vi "test8-AsteriskWildcardStatusRegistration.vi"(8 "error in (no error)":errorcluster, 11 "TestCase in":refnum<class "testcase-CSMStatusStateRegisterUnregister.lvclass">) -> (0 "error out":errorcluster, 3 "TestCase out":refnum<class "testcase-CSMStatusStateRegisterUnregister.lvclass">)   [LabVIEW 2017, in "testcase-CSMStatusStateRegisterUnregister.lvclass"]
uses:
  testcase-CSMStatusStateRegisterUnregister.lvclass
  0c20cacf-7d77-4f8e-aec5-f22e7d09936d.vi
  26de337d-8090-412f-9da5-e117a55d4726.vi
  de10340a-d592-45ad-b055-7fa7b377c551.vi
  e3eae2f8-d8ce-4adb-8167-9a417250fce1.vi
  a4d00e00-a9ed-4631-bf53-269bf71f16fc.vi
  src/user.lib/_NEVSTOP/Communicable State Machine(CSM)/AdvanceAPI/CSM - Revert Arguments-Safe String.vi
  src/user.lib/_NEVSTOP/Communicable State Machine(CSM)/AdvanceAPI/CSM - Make String Arguments Safe.vi
  src/user.lib/_NEVSTOP/Communicable State Machine(CSM)/AdvanceAPI/CSM - Break Down Multiple States String.vi
  src/user.lib/_NEVSTOP/Communicable State Machine(CSM)/AdvanceAPI/CSM - Compact Multiple States.vi
  src/user.lib/_NEVSTOP/Communicable State Machine(CSM)/AdvanceAPI/CSM - Keywords.vi
  src/user.lib/_NEVSTOP/Communicable State Machine(CSM)/_Shared/Trim Single-line Text.vi
  src/user.lib/_NEVSTOP/Communicable State Machine(CSM)/AdvanceAPI/CSM - Set Module Attribute.vi
  src/user.lib/_NEVSTOP/Communicable State Machine(CSM)/AdvanceAPI/CSM - Get Module Attribute.vi
  <vilib>/addons/_JKI Toolkits/VI Tester/TestCase.llb/TestCase.lvclass
  src/user.lib/_NEVSTOP/Communicable State Machine(CSM)/Communicable State Machine.lvlib
  C:/Program Files (x86)/National Instruments/LabVIEW 2017/vi.lib/addons/_JKI Toolkits/VI Tester/TestCase.llb/TestCase.lvclass
panel:
  out "error out 2":errorcluster
  out "Execution Times":i32
  out "State History":string
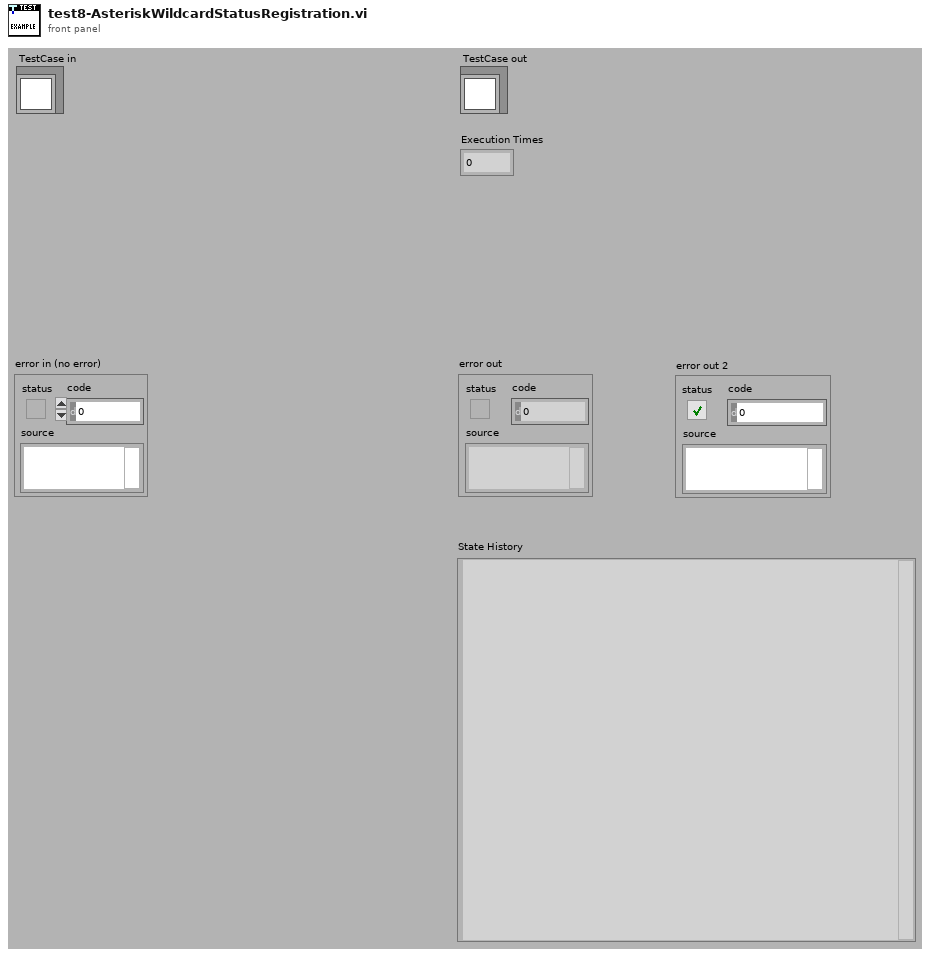
[diagram p1: front panel]
types:
  T1 = enum32{"Invalid", "Standard", "Closed", "Hidden", "Minimized", "Maximized"}
  T2 = enum32{"invalid app kind", "Development System", "Run Time System", "Student Edition", "Embedded LabVIEW", "Evaluation", "Custom"}
  T3 = typedef "Communicable State Machine.lvlib/_CSM_Response Source Message.ctl" = cluster{"‘State":string, "’Arguments":string, "’Error":errorcluster}
  T4 = cluster{"Current VI Reference":refnum<vi>, "Close Panel on Exit?":bool}
  T5 = cluster{"Core":cluster{"Current VI Reference":refnum<vi>, "Close Panel on Exit?":bool}, "Your Boolean data":bool, "Your string data":string, "TestData":i32}
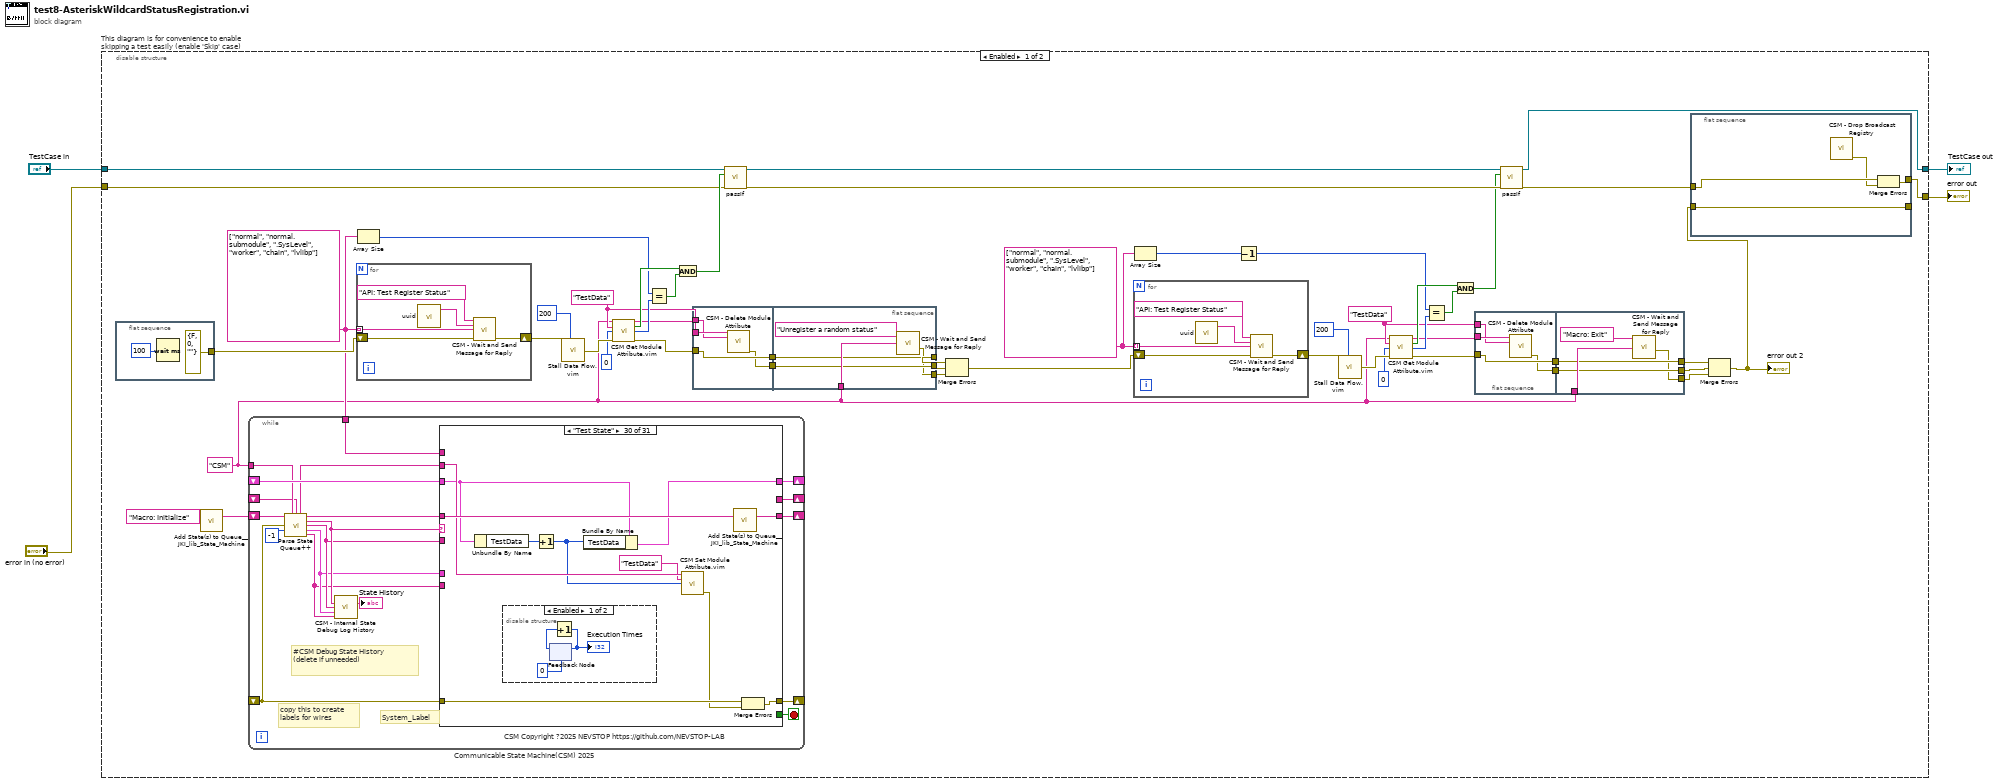
[diagram p0: block diagram]
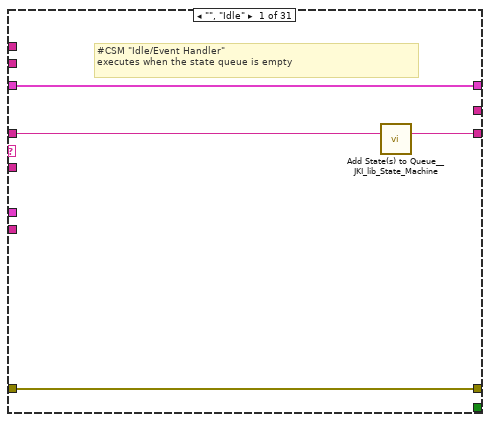
[diagram p2: hidden frame]
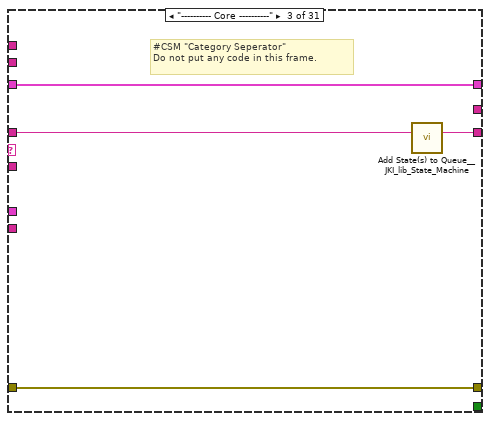
[diagram p4: hidden frame]
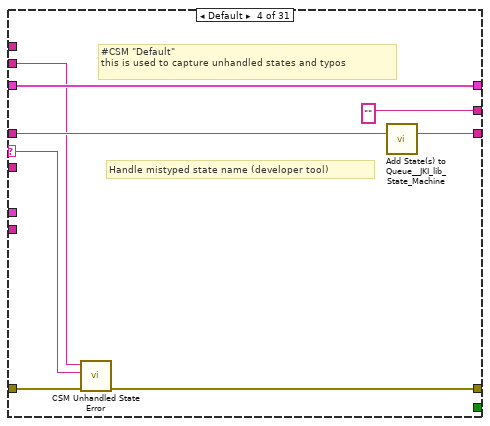
[diagram p5: hidden frame]
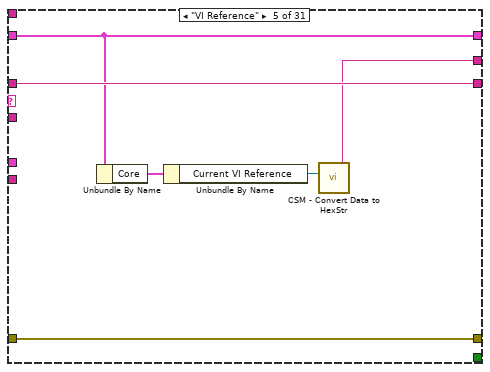
[diagram p6: hidden frame]
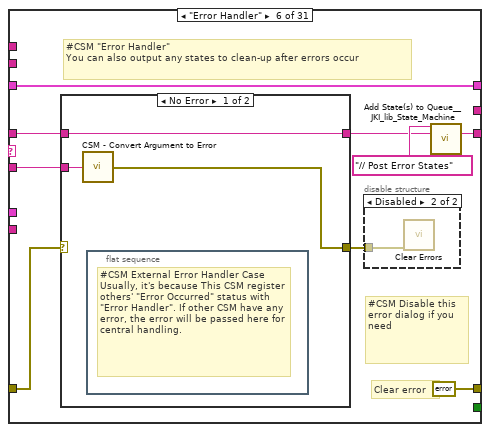
[diagram p7: hidden frame]
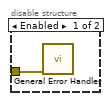
[diagram p8: hidden frame]
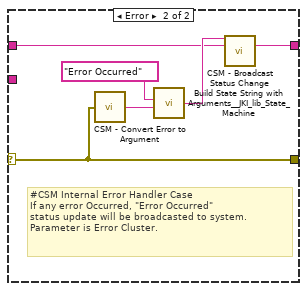
[diagram p9: hidden frame]
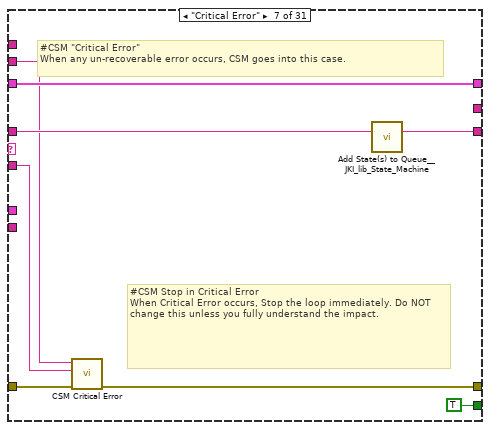
[diagram p10: hidden frame]
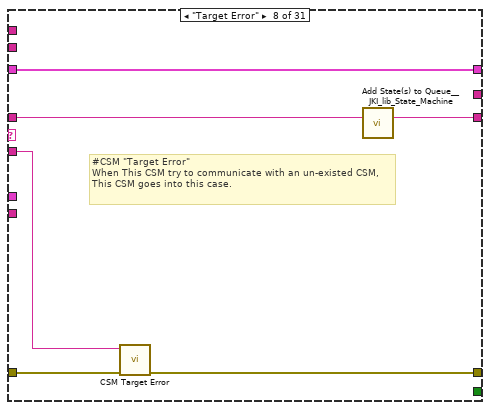
[diagram p11: hidden frame]
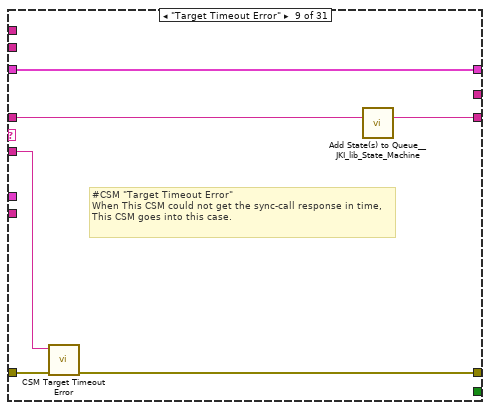
[diagram p12: hidden frame]
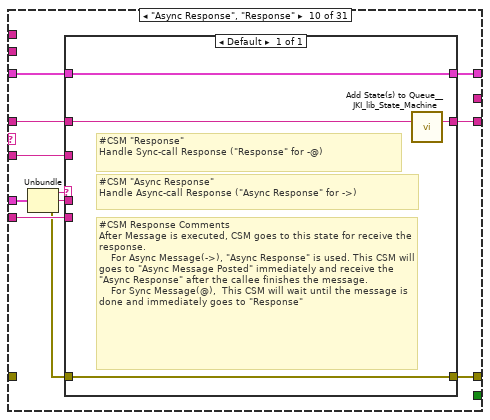
[diagram p13: hidden frame]
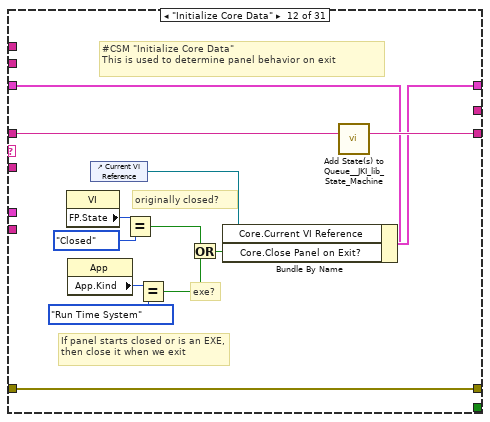
[diagram p15: hidden frame]
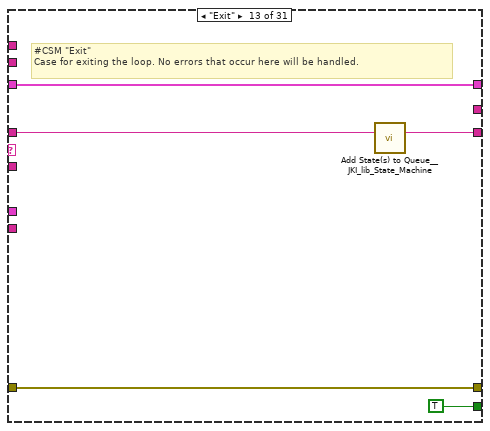
[diagram p16: hidden frame]
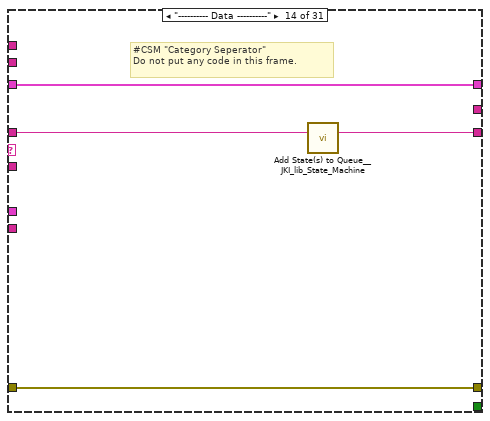
[diagram p17: hidden frame]
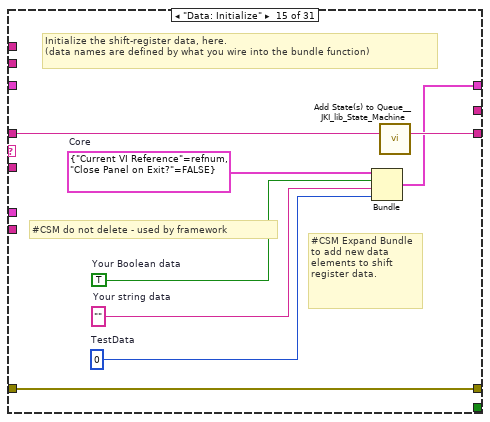
[diagram p18: hidden frame]
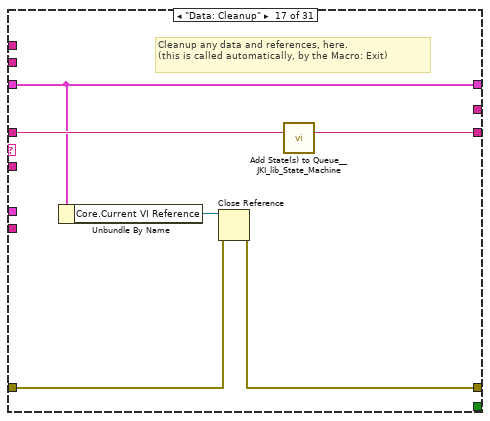
[diagram p20: hidden frame]
diagram:
  n1 = disable-structure "This diagram is for convenience to enable skipping a test easily (enable 'Skip' case)" shown="Enabled" {
    disable-tunnel: "TestCase in" -> [w41 w408]
    disable-tunnel: [w16 w406] -> w1
    disable-tunnel: [w52 w407] -> w3
    disable-tunnel: "error in (no error)" -> [w40 w405]
    frame Enabled {
      w12 = "TestData" ("Attribute")
      w23 = string[] ["normal", "normal.submodule", ".SysLevel", "worker", "chain", "lvlibp"]
      w38 = "TestData" ("Attribute")
      w10 = "CSM" ("Name (\"\" to Use UUID)")
      w31 = string[] ["normal", "normal.submodule", ".SysLevel", "worker", "chain", "lvlibp"]
      n2 = flat-sequence {
        tunnel: [errorcluster {"status"=FALSE, "code"=0, "source"=""} ("error in (no error)")] -> w51
        frame #0 {
          n3 = Wait (ms)(milliseconds to wait=u32 100) -> ()  [unwired: 1 out]
        }
      }
      n4 = call <vilib>:"Add State(s) to Queue__JKI_lib_State_Machine.vi"("State(s) in (\"\")"="Macro: Initialize" ("Init State(\"Macro: Initialize\")")) -> ("States Out"=w53:string)  [unwired: 14 in]
      n5 = while "Communicable State Machine(CSM) 2025" {
        shift-right: [w97] -> _
        shift-left: _ -> [w96]
        shift-right: [w100] -> _
        shift-left: _ -> [w95]
        shift-right: [w99] -> _
        shift-left: w53 -> [w101]
        tunnel: w10 -> [w93]
        shift-right: [w94] -> _
        shift-left: _ -> [w87]
        tunnel: w31 -> [w84]
        stop <- w98 stop-if-true
        # "#CSM Debug State History\n(delete if unneeded)"
        # "copy this to create labels for wires"
        # "System_Label"
        # "CSM Copyright ?2025 NEVSTOP https://github.com/NEVSTOP-LAB"
        n6 = call "Parse State Queue++.vi"("State Queue"=w101, "Name (\"\" to Use UUID)"=w93, "Response Arguments"=w87, "Previous Error"=w95, "Dequeue (1 ms)"=-1 ("Timeout")) -> ("Name Used"=w88:string, "Remaining States"=w102:string, "Current State"=w92:string, "Arguments"=w91:string, "Additional Information"=w90:T3, "Source CSM"=w89:string)  [unwired: 5 in]
        n7 = call "CSM - Internal State Debug Log History.vi"("State"=w92, "Arguments (\"\")"=w91, ">> Response Source Message >>"=w90, "Source (\"\")"=w89) -> ("Debug Log"=→"State History":string)  [unwired: 11 in]
        n8 = case shown="\"Test State\"" w92 {
          selector: w92 -> [_ _ _ w116 _ _ _ _ _ _ _ _ _ _ _ _ _ _ _ _ _ _ _ _ _ _ _ _ _ _ _]
          tunnel: w102 -> [w103 w108 w113 w120 w126 w132 w153 w159 w165 w173 w184 w198 w203 w207 w215 w217 w224 w228 w232 w238 w253 w322 w333 w346 w348 w352 w357 w364 w368 w379 w399]
          tunnel: w91 -> [_ _ _ _ _ w131 w149 w158 w163 w172 _ _ _ _ _ _ _ _ _ w233 w247 _ _ _ _ _ w355 _ _ _ _]
          tunnel: w96 -> [w104 w107 w110 w118 w125 w135 w154 w160 w166 w175 w183 w191 w201 w204 _ w216 w219 w225 w230 w236 w249 w319 w330 w343 w347 w351 w356 w361 w365 w371 w385]
          tunnel: [w105 w109 w111 w114 w127 errorcluster {"status"=FALSE, "code"=0, "source"=""} ("error out") w150 w156 w162 w178 w185 w195 w200 w205 w212 w218 w220 w226 w229 w234 w250 w320 w324 w335 w349 w353 w358 w362 w366 w373 w387] -> w100
          tunnel: w95 -> [w105 w109 w111 w121 w127 w133 w155 w157 w164 _ w185 w195 w200 w205 w212 w218 w221 w226 w229 w235 w251 w320 w331 w344 w349 w353 w358 w362 w366 w377 w397]
          tunnel: [w106 w108 w112 w119 w126 w128 w152 w161 w167 w174 w184 w197 w202 w206 w214 w217 w223 w227 w231 w237 w252 w321 w332 w345 w348 w352 w357 w363 w367 w378 w398] -> w99
          tunnel: [_ _ _ _ _ _ TRUE _ _ _ _ _ TRUE _ _ _ _ _ _ _ _ _ _ _ _ _ _ _ _ _ _] -> w98
          tunnel: [w104 w107 w110 w118 w125 w135 w154 w160 w166 w176 w183 w196 w201 w204 w213 w216 w219 w225 w230 w236 w249 w319 w330 w343 w347 w351 w356 w361 w365 w375 w383] -> w97
          tunnel: w89 -> [_ _ _ _ _ _ _ _ _ w170 _ _ _ _ _ _ _ _ _ _ _ _ _ _ _ _ _ _ _ _ _]
          tunnel: w90 -> [_ _ _ _ _ _ _ _ _ w177 _ _ _ _ _ _ _ _ _ _ _ _ _ _ _ _ _ _ _ _ _]
          tunnel: [_ _ _ "" w122 _ _ _ _ _ _ _ _ _ _ _ _ _ _ _ _ _ _ _ _ "API1 Response" w354 _ _ _ _] -> w94
          tunnel: w88 -> [_ _ _ w115 _ _ w148 _ _ _ _ _ _ _ _ _ _ _ _ _ _ _ w325 w337 _ _ _ _ _ w374 w394]
          tunnel: w84 -> [_ _ _ _ _ _ _ _ _ _ _ _ _ _ _ _ _ _ _ _ _ _ _ _ _ _ _ _ _ _ w390]
          frame "", "Idle" {
            # "#CSM \"Idle/Event Handler\"\nexecutes when the state queue is empty"
            n9 = call <vilib>:"Add State(s) to Queue__JKI_lib_State_Machine.vi"("State(s) in (\"\")"=w103) -> ("States Out"=w106:string)  [unwired: 14 in]
          }
          frame "CSM Documentation" {
            # "#CSM README FIRST\n\nCommunicable State Machine(CSM) is a LabVIEW application framework that builds upon JKI State Machine(JKISM). It follows the pattern of JKISM and extends the keywords to describe message communication between modules, including concepts such as Sync-Message, Async-Message, Subscription/Unsubscription of status - essential elements for creating reusable code modules. For more information, please visit the CSM wiki: https://nevstop-lab.github.io/CSM-Wiki/\n\nFor instructions on JKI State Machine, visit: http://jki.net/state-machine/\nFor information about CSM, visit: https://github.com/NEVSTOP-LAB"
            # "#CSM \"Documentation\"\nCase for holding CSM Documenation"
          }
          frame "---------- Core ----------" {
            # "#CSM \"Category Seperator\"\nDo not put any code in this frame."
            n10 = call <vilib>:"Add State(s) to Queue__JKI_lib_State_Machine.vi"("State(s) in (\"\")"=w113) -> ("States Out"=w112:string)  [unwired: 14 in]
          }
          frame Default {
            # "#CSM \"Default\"\nthis is used to capture unhandled states and typos"
            # "Handle mistyped state name (developer tool)"
            n11 = call "CSM Unhandled State Error.vi"("error in (no error)"=w121, "Undefined State"=w116, "CSM Name"=w115) -> ("error out"=w114:errorcluster)  [unwired: 8 in]
            n12 = call <vilib>:"Add State(s) to Queue__JKI_lib_State_Machine.vi"("State(s) in (\"\")"=w120) -> ("States Out"=w119:string)  [unwired: 14 in]
          }
          frame "VI Reference" {
            n13 = Unbundle By Name(w125) -> ("Core"=w124:T4)
            n14 = Unbundle By Name(w124) -> ("Current VI Reference"=w123:refnum<vi>)
            n15 = call "CSM - Convert Data to HexStr.vi"("Variant"=w123) -> ("HEX String (0-9,A-F)"=w122:string)  [unwired: 8 in]
          }
          frame "Error Handler" {
            # "#CSM Disable this error dialog if you need"
            # "#CSM \"Error Handler\"\nYou can also output any states to clean-up after errors occur"
            # "Clear error"
            n16 = case shown="No Error" w133 {
              selector: w133 -> [_ w142]
              tunnel: [w141 w144] -> w129
              tunnel: w132 -> [w141 w143]
              tunnel: w131 -> [w140 _]
              tunnel: [w139 w142] -> w134
              frame No Error {
                n17 = call "CSM - Convert Argument to Error.vi"("Argument"=w140) -> ("Error"=w139:errorcluster)  [unwired: 4 in]
                n18 = flat-sequence {
                  frame #0 {
                    # "#CSM External Error Handler Case\nUsually, it's because This CSM register others' \"Error Occurred\" status with \"Error Handler\". If other CSM have any error, the error will be passed here for central handling."
                  }
                }
              }
              frame Error {
                # "#CSM Internal Error Handler Case \nIf any error Occurred, \"Error Occurred\" \nstatus update will be broadcasted to system.\nParameter is Error Cluster."
                n19 = call "CSM - Convert Error to Argument.vi"("Error"=w142) -> ("Argument"=w146:string)  [unwired: 4 in]
                n20 = call <vilib>:"Build State String with Arguments__JKI_lib_State_Machine.vi"("Arguments (\"\")"=w146, "State"="Error Occurred" ("Status with Arguments")) -> ("State with Arguments"=w145:string)  [unwired: 4 in]
                n21 = call "CSM - Broadcast Status Change.vi"("Status With Arguments"=w145, "State Queue"=w143) -> ("Remaining States"=w144:string)  [unwired: 13 in]
              }
            }
            n22 = disable-structure shown="Disabled" {
              disable-tunnel: w134 -> [w137 w138]
              frame Enabled {
                n23 = call <vilib>:"General Error Handler.vi"("error in (no error)"=w137) -> ()  [unwired: 10 in, 5 out]
              }
              frame Disabled {
                n24 = call <vilib>:"Clear Errors.vi"("error in (no error)"=w138) -> ()  [unwired: 5 in, 2 out]
              }
            }
            n25 = call <vilib>:"Add State(s) to Queue__JKI_lib_State_Machine.vi"("State(s) in Front (\"\")"="// Post Error States", "State(s) in (\"\")"=w129) -> ("States Out"=w128:string)  [unwired: 13 in]
          }
          frame "Critical Error" {
            # "#CSM Stop in Critical Error\nWhen Critical Error occurs, Stop the loop immediately. Do NOT change this unless you fully understand the impact."
            # "#CSM \"Critical Error\"\nWhen any un-recoverable error occurs, CSM goes into this case."
            n26 = call "CSM Critical Error.vi"("error in (no error)"=w155, "Arugments (As Reason)"=w149, "CSM Name"=w148) -> ("error out"=w150:errorcluster)  [unwired: 8 in]
            n27 = call <vilib>:"Add State(s) to Queue__JKI_lib_State_Machine.vi"("State(s) in (\"\")"=w153) -> ("States Out"=w152:string)  [unwired: 14 in]
          }
          frame "Target Error" {
            # "#CSM \"Target Error\"\nWhen This CSM try to communicate with an un-existed CSM, This CSM goes into this case."
            n28 = call "CSM Target Error.vi"("error in (no error)"=w157, "Arguments (As CSM Name)"=w158) -> ("error out"=w156:errorcluster)  [unwired: 9 in]
            n29 = call <vilib>:"Add State(s) to Queue__JKI_lib_State_Machine.vi"("State(s) in (\"\")"=w159) -> ("States Out"=w161:string)  [unwired: 14 in]
          }
          frame "Target Timeout Error" {
            # "#CSM \"Target Timeout Error\"\nWhen This CSM could not get the sync-call response in time, This CSM goes into this case."
            n30 = call "CSM Target Timeout Error.vi"("error in (no error)"=w164, "Arguments (As CSM Name)"=w163) -> ("error out"=w162:errorcluster)  [unwired: 9 in]
            n31 = call <vilib>:"Add State(s) to Queue__JKI_lib_State_Machine.vi"("State(s) in (\"\")"=w165) -> ("States Out"=w167:string)  [unwired: 14 in]
          }
          frame "Async Response", "Response" {
            n32 = Unbundle(w177) -> ("‘State"=w171:string, "’Arguments"=w169:string, "’Error"=w168:errorcluster)
            n33 = case shown="Default" w171 {
              tunnel: [w182] -> w178
              tunnel: w168 -> [w182]
              tunnel: [w181] -> w176
              tunnel: w175 -> [w181]
              tunnel: [w179] -> w174
              tunnel: w173 -> [w180]
              tunnel: w172 -> [_]
              tunnel: w170 -> [_]
              tunnel: w169 -> [_]
              frame Default {
                # "#CSM Response Comments\nAfter Message is executed, CSM goes to this state for receive the response.\n    For Async Message(->), \"Async Response\" is used. This CSM will goes to \"Async Message Posted\" immediately and receive the \"Async Response\" after the callee finishes the message.\n    For Sync Message(@),  This CSM will wait until the message is done and immediately goes to \"Response\""
                # "#CSM \"Async Response\"\nHandle Async-call Response (\"Async Response\" for ->)"
                # "#CSM \"Response\"\nHandle Sync-call Response (\"Response\" for -@)"
                n34 = call <vilib>:"Add State(s) to Queue__JKI_lib_State_Machine.vi"("State(s) in (\"\")"=w180) -> ("States Out"=w179:string)  [unwired: 14 in]
              }
            }
          }
          frame "Async Message Posted" {
            # "#CSM \"Async Message Posted\"\nAfter Async Message is posted (-> or ->| ), CSM goes to this state for post-action.\nYou can use Argument - State to tell which Async Message is called."
          }
          frame "Initialize Core Data" {
            # "#CSM \"Initialize Core Data\"\nThis is used to determine panel behavior on exit"
            # "originally closed?"
            # "exe?"
            # "If panel starts closed or is an EXE, then close it when we exit"
            n35 = property class="VI"() -> ("FP.State"=w188:T1)  [unwired: 2 in, 2 out]
            n36 = property class="App"() -> ("App.Kind"=w194:T2)  [unwired: 2 in, 2 out]
            n37 = control-ref of="Current VI Reference"() -> (w189:refnum<vi>)
            n38 = Equal?(x=w188, y=T1."Closed" ("Front Panel Window:State")) -> (x = y?=w186:bool)
            n39 = Equal?(x=w194, y=T2."Run Time System" ("Application:Kind")) -> (x = y?=w192:bool)
            n40 = Or(x=w186, y=w192) -> (x .or. y?=w190:bool)
            n41 = Bundle By Name(cluster=w191, "Core.Current VI Reference"=w189, "Core.Close Panel on Exit?"=w190) -> (w196:T5)
            n42 = call <vilib>:"Add State(s) to Queue__JKI_lib_State_Machine.vi"("State(s) in (\"\")"=w198) -> ("States Out"=w197:string)  [unwired: 14 in]
          }
          frame "Exit" {
            # "#CSM \"Exit\"\nCase for exiting the loop. No errors that occur here will be handled."
            n43 = call <vilib>:"Add State(s) to Queue__JKI_lib_State_Machine.vi"("State(s) in (\"\")"=w203) -> ("States Out"=w202:string)  [unwired: 14 in]
          }
          frame "---------- Data ----------" {
            # "#CSM \"Category Seperator\"\nDo not put any code in this frame."
            n44 = call <vilib>:"Add State(s) to Queue__JKI_lib_State_Machine.vi"("State(s) in (\"\")"=w207) -> ("States Out"=w206:string)  [unwired: 14 in]
          }
          frame "Data: Initialize" {
            w208 = 0  # TestData
            w209 = T4 {"Current VI Reference"=refnum, "Close Panel on Exit?"=FALSE}  # Core
            w211 = TRUE  # Your Boolean data
            w210 = ""  # Your string data
            # "#CSM do not delete - used by framework"
            # "#CSM Expand Bundle to add new data elements to shift register data."
            # "Initialize the shift-register data, here.\n(data names are defined by what you wire into the bundle function)"
            n45 = Bundle("Core"=w209, "Your Boolean data"=w211, "Your string data"=w210, "TestData"=w208) -> (w213:T5)  [unwired: 1 in]
            n46 = call <vilib>:"Add State(s) to Queue__JKI_lib_State_Machine.vi"("State(s) in (\"\")"=w215) -> ("States Out"=w214:string)  [unwired: 14 in]
          }
          frame "Data: Update Indicators" {
          }
          frame "Data: Cleanup" {
            # "Cleanup any data and references, here.\n(this is called automatically, by the Macro: Exit)"
            n47 = Unbundle By Name(w219) -> ("Core.Current VI Reference"=w222:refnum<vi>)
            n48 = Close Reference(reference=w222, error in (no error)=w221) -> (error out=w220:errorcluster)
            n49 = call <vilib>:"Add State(s) to Queue__JKI_lib_State_Machine.vi"("State(s) in (\"\")"=w224) -> ("States Out"=w223:string)  [unwired: 14 in]
          }
          frame "---------- UI ----------" {
            # "#CSM \"Category Seperator\"\nDo not put any code in this frame."
            n50 = call <vilib>:"Add State(s) to Queue__JKI_lib_State_Machine.vi"("State(s) in (\"\")"=w228) -> ("States Out"=w227:string)  [unwired: 14 in]
          }
          frame "UI: Initialize" {
            # "#CSM \"UI: Initialize\"\nInitialize the User Interface, here.\n(this is called automatically, by the Macro: Init)"
            n51 = call <vilib>:"Add State(s) to Queue__JKI_lib_State_Machine.vi"("State(s) in (\"\")"=w232) -> ("States Out"=w231:string)  [unwired: 14 in]
          }
          frame "UI: Cursor Set" {
            # "#CSM \"UI: Cursor Set\"\nSet and Unset Cursor Busy.\n(Usage: \"UI: Cursor Set >> Busy|Idle\")"
            # "Argument"
            n52 = disable-structure shown="TARGET_TYPE!=Windows" {
              disable-tunnel: w235 -> [w241 w246]
              disable-tunnel: [w240 w246] -> w234
              disable-tunnel: w233 -> [w239 _]
              frame condition #0 (active) {
                n53 = case shown="\"Idle\", Default" w239 {
                  tunnel: w241 -> [w243 w245]
                  tunnel: [w242 w244] -> w240
                  frame "Idle", Default {
                    n54 = call <vilib>:"Unset Busy.vi"("error in (no error)"=w243) -> ("error out"=w242:errorcluster)  [unwired: 10 in]
                  }
                  frame "Busy" {
                    n55 = call <vilib>:"Set Busy.vi"("error in (no error)"=w245) -> ("error out"=w244:errorcluster)  [unwired: 9 in, 1 out]
                  }
                }
              }
              frame condition #1 {
              }
            }
            n56 = call <vilib>:"Add State(s) to Queue__JKI_lib_State_Machine.vi"("State(s) in (\"\")"=w238) -> ("States Out"=w237:string)  [unwired: 14 in]
          }
          frame "UI: Front Panel State" {
            # "#CSM \"UI: Front Panel State\"\nSet Front Panel Open or Closed\n(Usage: \"UI: Front Panel State >> Open|Close\")"
            # "Argument"
            n57 = Unbundle By Name(w249) -> ("Core.Current VI Reference"=w248:refnum<vi>)
            n58 = call <vilib>:"Add State(s) to Queue__JKI_lib_State_Machine.vi"("State(s) in (\"\")"=w253) -> ("States Out"=w252:string)  [unwired: 14 in]
            n59 = case shown="\"Close\", \"Closed\"" w247 {
              tunnel: w251 -> [w259 w274 w285 w298 w311]
              tunnel: [w261 w275 w287 w300 w313] -> w250
              tunnel: w248 -> [w260 w272 w286 w299 w312]
              frame "Open", "Standard", Default {
                w254 = T1."Standard" ("State")
                n60 = property class="VI"(reference=w260, error in=w259) -> (reference out=w257:refnum<vi>, error out=w258:errorcluster, "FP.State"=w256:T1)
                n61 = Not Equal?(x=w256, y=w254) -> (x != y?=w255:bool)
                n62 = case shown="True" w255 {
                  tunnel: [w265 w267] -> w261
                  tunnel: w258 -> [w264 w267]
                  tunnel: w257 -> [w263 _]
                  tunnel: w254 -> [w262 _]
                  frame True {
                    n63 = invoke class="VI" method="FP.Open"(reference=w263, error in=w264, "Activate"=TRUE, "State"=w262) -> (error out=w265:errorcluster)  [unwired: 1 in, 4 out]
                  }
                  frame False {
                  }
                }
              }
              frame "Close", "Closed" {
                n64 = property class="VI"(reference=w272, error in=w274) -> (reference out=w271:refnum<vi>, error out=w273:errorcluster, "FP.State"=w269:T1)
                n65 = Not Equal?(x=w269, y=T1."Closed" ("Front Panel Window:State")) -> (x != y?=w268:bool)
                n66 = case shown="False" w268 {
                  tunnel: [w276 w279] -> w275
                  tunnel: w273 -> [w276 w278]
                  tunnel: w271 -> [_ w277]
                  frame False {
                  }
                  frame True {
                    n67 = invoke class="VI" method="FP.Close"(reference=w277, error in=w278) -> (error out=w279:errorcluster)  [unwired: 1 in, 2 out]
                  }
                }
              }
              frame "Hidden", "Hide" {
                w280 = T1."Hidden" ("State")
                n68 = property class="VI"(reference=w286, error in=w285) -> (reference out=w283:refnum<vi>, error out=w284:errorcluster, "FP.State"=w282:T1)
                n69 = Not Equal?(x=w282, y=w280) -> (x != y?=w281:bool)
                n70 = case shown="True" w281 {
                  tunnel: [w291 w292] -> w287
                  tunnel: w284 -> [w290 w292]
                  tunnel: w283 -> [w289 _]
                  tunnel: w280 -> [w288 _]
                  frame True {
                    n71 = invoke class="VI" method="FP.Open"(reference=w289, error in=w290, "State"=w288) -> (error out=w291:errorcluster)  [unwired: 2 in, 4 out]
                  }
                  frame False {
                  }
                }
              }
              frame "Minimize", "Minimized" {
                w293 = T1."Minimized" ("State")
                n72 = property class="VI"(reference=w299, error in=w298) -> (reference out=w296:refnum<vi>, error out=w297:errorcluster, "FP.State"=w295:T1)
                n73 = Not Equal?(x=w295, y=w293) -> (x != y?=w294:bool)
                n74 = case shown="True" w294 {
                  tunnel: [w304 w305] -> w300
                  tunnel: w297 -> [w303 w305]
                  tunnel: w296 -> [w302 _]
                  tunnel: w293 -> [w301 _]
                  frame True {
                    n75 = invoke class="VI" method="FP.Open"(reference=w302, error in=w303, "State"=w301) -> (error out=w304:errorcluster)  [unwired: 2 in, 4 out]
                  }
                  frame False {
                  }
                }
              }
              frame "Maximize", "Maximized" {
                w306 = T1."Maximized" ("State")
                n76 = property class="VI"(reference=w312, error in=w311) -> (reference out=w309:refnum<vi>, error out=w310:errorcluster, "FP.State"=w308:T1)
                n77 = Not Equal?(x=w308, y=w306) -> (x != y?=w307:bool)
                n78 = case shown="True" w307 {
                  tunnel: [w317 w318] -> w313
                  tunnel: w310 -> [w316 w318]
                  tunnel: w309 -> [w315 _]
                  tunnel: w306 -> [w314 _]
                  frame True {
                    n79 = invoke class="VI" method="FP.Open"(reference=w315, error in=w316, "State"=w314) -> (error out=w317:errorcluster)  [unwired: 2 in, 4 out]
                  }
                  frame False {
                  }
                }
              }
            }
          }
          frame "---------- Macro ----------" {
            # "#CSM \"Category Seperator\"\nDo not put any code in this frame."
            n80 = call <vilib>:"Add State(s) to Queue__JKI_lib_State_Machine.vi"("State(s) in (\"\")"=w322) -> ("States Out"=w321:string)  [unwired: 14 in]
          }
          frame "Macro: Initialize" {
            # "#CSM \"Macro: Initialize\"\nInitialization Macro (This is called once, when the VI starts)"
            n81 = call "CSM - Register Broadcast.vi"("CSM Name"=w325, "Source CSM Name (* as Default)"="*", "Trigger"="Test Status" ("Status"), "API (If \"\", Same as Trigger)"="Test State" ("Response Message (If \"\", Same as Source Message)")) -> ("error out"=w323:errorcluster)  [unwired: 10 in, 1 out]
            n82 = Merge Errors(w323, w331) -> (w324:errorcluster)
            n83 = call <vilib>:"Add State(s) to Queue__JKI_lib_State_Machine.vi"("State(s) in Front (\"\")"="Data: Initialize\nInitialize Core Data\nData: Update Indicators", "State(s) in (\"\")"=w333) -> ("States Out"=w332:string)  [unwired: 13 in]
          }
          frame "Macro: Exit" {
            # "#CSM \"Macro: Exit\"\nExit Macro (This is called once, when the VI exits)"
            n84 = call "CSM - Unregister Broadcast.vi"("CSM Name"=w337, "Source CSM Name (* as Default)"="*", "Trigger"="Test Status" ("Status"), "API (\"*\" as Default)"="Test State" ("Response Message (If \"\", Same as Source Message)")) -> ("error out"=w334:errorcluster)  [unwired: 10 in, 1 out]
            n85 = call <vilib>:"Add State(s) to Queue__JKI_lib_State_Machine.vi"("State(s) in Front (\"\")"="//Exit Sub-Modules ", "State(s) at Back (\"\")"="Data: Cleanup\nExit") -> ("States Out"=w341:string)  [unwired: 13 in]
            n86 = Merge Errors(w334, w344) -> (w335:errorcluster)
            n87 = call <vilib>:"Add State(s) to Queue__JKI_lib_State_Machine.vi"("State(s) in Front (\"\")"=w341, "State(s) in (\"\")"=w346) -> ("States Out"=w345:string)  [unwired: 13 in]
          }
          frame "---------- API ----------" {
            # "#CSM \"Category Seperator\"\nDo not put any code in this frame."
          }
          frame "API: API1" {
            # "#CSM API Example\nCopy/Rename this case for your own API"
            # "#CSM Response\nConnect this to return the response of your API"
            # "#CSM >> Msg/Rep's CSM >>\nIf you need to tell who triggered this state , use this string. If it's this case itself, this string is \"\"."
            # "#CSM >> Arguments >>\nDeal with the parameter if any"
          }
          frame "API: API2" {
            # "#CSM API Example\nCopy/Rename this case for your own API"
            # "unpack Hex String  to Variant\nif complex parameter is needed."
            n88 = call "CSM - Convert HexStr to Data.vi"("HEX String"=w355) -> ()  [unwired: 7 in, 2 out]
            n89 = disable-structure shown="Disabled" {
              disable-tunnel: [w359 "API2 Response"] -> w354
              frame Disabled {
                # "pack variant to hexstr \nif complex response is needed."
                # "complex Response"
                n90 = call "CSM - Convert Data to HexStr.vi"() -> ("HEX String (0-9,A-F)"=w359:string)  [unwired: 9 in]
              }
              frame Enabled {
              }
            }
          }
          frame "---------- Action ----------" {
            # "#CSM \"Category Seperator\"\nDo not put any code in this frame."
            n91 = call <vilib>:"Add State(s) to Queue__JKI_lib_State_Machine.vi"("State(s) in (\"\")"=w364) -> ("States Out"=w363:string)  [unwired: 14 in]
          }
          frame "Action: action1" {
            # "#CSM \"Internal State\"\nThis category is used for holding internal states"
            n92 = call <vilib>:"Add State(s) to Queue__JKI_lib_State_Machine.vi"("State(s) in (\"\")"=w368) -> ("States Out"=w367:string)  [unwired: 14 in]
          }
          frame "Test State" {
            n93 = Unbundle By Name(w371) -> ("TestData"=w376:i32)
            n94 = disable-structure shown="Enabled" {
              frame Enabled {
                n95 = feedback #1(0 ("y")) -> (w381:i32)
                n96 = Increment(x=w381) -> (x+1=w380:i32)
                "Execution Times" <- w380
                n97 = feedback-in #1(w380) -> ()
              }
              frame Disabled {
              }
            }
            n98 = Increment(x=w376) -> (x+1=w369:i32)
            n99 = Bundle By Name(cluster=w371, "TestData"=w369) -> (w375:T5)
            n100 = call "CSM Set Module Attribute.vim"("CSM Name"=w374, "Attribute"="TestData", "Value"=w369) -> ("error out"=w372:errorcluster)  [unwired: 9 in, 3 out]
            n101 = call <vilib>:"Add State(s) to Queue__JKI_lib_State_Machine.vi"("State(s) in (\"\")"=w379) -> ("States Out"=w378:string)  [unwired: 14 in]
            n102 = Merge Errors(w377, w372) -> (w373:errorcluster)
          }
          frame "Unregister a random status" {
            n103 = Random Number (0-1)() -> (number: 0 to 1=w392:dbl)
            n104 = Array Size(array=w390) -> (size(s)=w393:i32)
            n105 = Multiply(x=w393, y=w392) -> (x*y=w391:dbl)
            n106 = Bundle By Name(cluster=w385, "TestData"=0) -> (w383:T5)
            n107 = Round Toward -Infinity(1:w391) -> (0:w389:dbl)
            n108 = Index Array(array=w390, index=w389) -> (element=w388:string)
            n109 = call "CSM - Unregister Broadcast.vi"("CSM Name"=w394, "Source CSM Name (* as Default)"=w388, "Trigger"="Test Status" ("Status"), "API (\"*\" as Default)"="Test State" ("Response Message (If \"\", Same as Source Message)")) -> ("error out"=w386:errorcluster)  [unwired: 10 in, 1 out]
            n110 = Merge Errors(w397, w386) -> (w387:errorcluster)
            n111 = call <vilib>:"Add State(s) to Queue__JKI_lib_State_Machine.vi"("State(s) in (\"\")"=w399) -> ("States Out"=w398:string)  [unwired: 14 in]
          }
        }
      }
      n112 = for {
        tunnel: w31 -> [w402] mode=indexing
        shift-right: [w401] -> w49
        shift-left: w51 -> [w400]
        n113 = call "uuid.vi"() -> ("UUID"=w403:string)  [unwired: 11 in]
        n114 = call "CSM - Wait and Send Message for Reply.vi"("State"="API: Test Register Status", "Arguments (\"\")"=w403, "Target Module"=w402, "Error In (No Error)"=w400) -> ("error out"=w401:errorcluster)  [unwired: 9 in, 2 out]
      }
      n115 = Array Size(array=w31) -> (size(s)=w44:i32)
      n116 = call "Stall Data Flow.vim"("value in"=w49, "milliseconds to wait"=u32 200) -> ("value out"=w48:errorcluster)  [unwired: 1 out]
      n117 = call "CSM Get Module Attribute.vim"("CSM Name"=w10, "Attribute"=w38, "Default Value (Empty Variant)"=0 ("x+1"), "Error In"=w48) -> ("CSM Name (Dup)"=w39:string, "Found"=w46:bool, "Value"=w45:i32, "error out"=w37:errorcluster)  [unwired: 7 in, 1 out]
      n118 = Equal?(x=w44, y=w45) -> (x = y?=w43:bool)
      n119 = And(x=w46, y=w43) -> (x .and. y?=w42:bool)
      n120 = flat-sequence {
        tunnel: w39 -> [w72]
        tunnel: w38 -> [w71]
        tunnel: w37 -> [w70]
        tunnel: [w70] -> w36
        tunnel: [w69] -> w35
        tunnel: w10 -> [w76]
        tunnel: w36 -> [w75]
        tunnel: w35 -> [w74]
        tunnel: [w75] -> w34
        tunnel: [w74] -> w33
        tunnel: [w73] -> w32
        frame #0 {
          n121 = call "CSM - Delete Module Attribute.vi"("CSM Name"=w72, "Attribute"=w71) -> ("error out"=w69:errorcluster)  [unwired: 10 in, 3 out]
        }
        frame #1 {
          n122 = call "CSM - Wait and Send Message for Reply.vi"("State"="Unregister a random status", "Target Module"=w76) -> ("error out"=w73:errorcluster)  [unwired: 11 in, 2 out]
        }
      }
      n123 = call-dynamic "passIf.vi"("error in (no error)"=w40, "pass"=w42, "TestCase in"=w41) -> ("error out"=w19:errorcluster, "TestCase out"=w17:refnum<class "testcase-CSMStatusStateRegisterUnregister.lvclass">)  [unwired: 7 in]
      n124 = Merge Errors(w34, w33, w32) -> (w22:errorcluster)
      n125 = for {
        tunnel: w23 -> [w66] mode=indexing
        shift-right: [w65] -> w29
        shift-left: w22 -> [w64]
        n126 = call "uuid.vi"() -> ("UUID"=w67:string)  [unwired: 11 in]
        n127 = call "CSM - Wait and Send Message for Reply.vi"("State"="API: Test Register Status", "Arguments (\"\")"=w67, "Target Module"=w66, "Error In (No Error)"=w64) -> ("error out"=w65:errorcluster)  [unwired: 9 in, 2 out]
      }
      n128 = Array Size(array=w23) -> (size(s)=w21:i32)
      n129 = Decrement(x=w21) -> (x-1=w20:i32)
      n130 = call "Stall Data Flow.vim"("value in"=w29, "milliseconds to wait"=u32 200) -> ("value out"=w28:errorcluster)  [unwired: 1 out]
      n131 = call "CSM Get Module Attribute.vim"("CSM Name"=w10, "Attribute"=w12, "Default Value (Empty Variant)"=0 ("x+1"), "Error In"=w28) -> ("CSM Name (Dup)"=w13:string, "Found"=w26:bool, "Value"=w25:i32, "error out"=w11:errorcluster)  [unwired: 7 in, 1 out]
      n132 = Equal?(x=w20, y=w25) -> (x = y?=w24:bool)
      n133 = And(x=w26, y=w24) -> (x .and. y?=w5:bool)
      n134 = flat-sequence {
        tunnel: w13 -> [w58]
        tunnel: w12 -> [w57]
        tunnel: w11 -> [w56]
        tunnel: [w56] -> w15
        tunnel: [w55] -> w14
        tunnel: w10 -> [w62]
        tunnel: w15 -> [w61]
        tunnel: w14 -> [w60]
        tunnel: [w61] -> w9
        tunnel: [w60] -> w8
        tunnel: [w59] -> w7
        frame #0 {
          n135 = call "CSM - Delete Module Attribute.vi"("CSM Name"=w58, "Attribute"=w57) -> ("error out"=w55:errorcluster)  [unwired: 10 in, 3 out]
        }
        frame #1 {
          n136 = call "CSM - Wait and Send Message for Reply.vi"("State"="Macro: Exit", "Target Module"=w62) -> ("error out"=w59:errorcluster)  [unwired: 11 in, 2 out]
        }
      }
      n137 = call-dynamic "passIf.vi"("error in (no error)"=w19, "pass"=w5, "TestCase in"=w17) -> ("error out"=w18:errorcluster, "TestCase out"=w16:refnum<class "testcase-CSMStatusStateRegisterUnregister.lvclass">)  [unwired: 7 in]
      n138 = flat-sequence {
        tunnel: [w83] -> w52
        tunnel: w18 -> [w82]
        tunnel: w6 -> [w81]
        tunnel: [w81] -> _
        frame #0 {
          n139 = call "CSM - Drop Broadcast Registry.vi"() -> ("error out"=w80:errorcluster)  [unwired: 15 in]
          n140 = Merge Errors(w82, w80) -> (w83:errorcluster)
        }
      }
      n141 = Merge Errors(w9, w8, w7) -> (w6:errorcluster)
      "error out 2" <- w6
    }
    frame Disabled {
      # "skip test result while test is under development"
      n142 = call <vilib>:"skip.vi"("error in (no error)"=w405, "TestCase in"=w408) -> ("error out"=w407:errorcluster, "TestCase out"=w406:refnum<class "testcase-CSMStatusStateRegisterUnregister.lvclass">)  [unwired: 8 in]
    }
  }
  "error out" <- w3
  "TestCase out" <- w1
